vi "VersionCheck.vi"(0 "Version":string, 1 "error in (no error)":errorcluster) -> (2 "Latest Version":string, 3 "outdated?":bool, 4 "error out":errorcluster)   [LabVIEW 2024]
uses:
  <vilib>/regexp/Match Regular Expression.xnode
panel:
  out "standard output":string
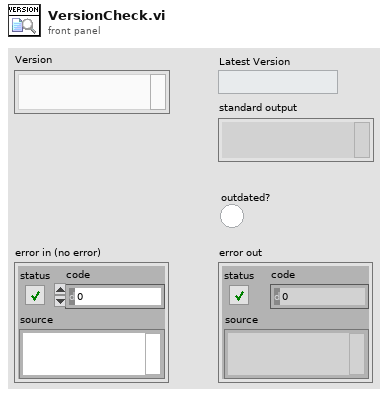
[diagram p1: front panel]
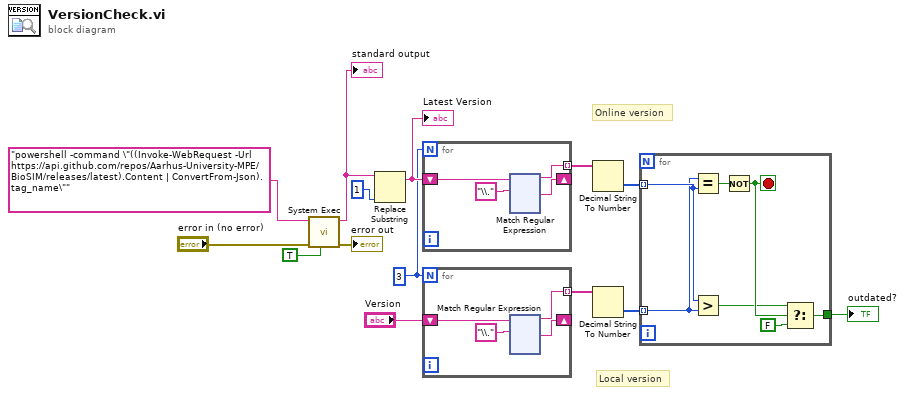
[diagram p0: block diagram]
diagram:
  w3 = 3
  # "Local version"
  # "Online version"
  n1 = call <vilib>:"System Exec.vi"("run minimized? (F)"=TRUE, "error in (no error)"="error in (no error)", "command line"="powershell -command \"((Invoke-WebRequest -Url https://api.github.com/repos/Aarhus-University-MPE/BioSIM/releases/latest).Content | ConvertFrom-Json).tag_name\"") -> ("error out"=→"error out":errorcluster, "standard output"=w12:string)  [unwired: 5 in, 2 out]
  "standard output" <- w12
  n2 = Replace Substring(2:1 ("length (len. of substring)"), 5:w12) -> (1:w10:string)  [unwired: 2 in, 1 out]
  "Latest Version" <- w10
  n3 = for {
    N: w3 -> [_]
    shift-right: [w16] -> _
    shift-left: w10 -> [w17]
    tunnel: [w15] -> w9 mode=indexing
    n4 = xnode "Match Regular Expression"("input string"=w17, "regular expression"="\\.") -> ("before match"=w15:string, "after match"=w16:string)  [unwired: 4 in, 3 out]
  }
  n5 = for {
    N: w3 -> [_]
    shift-right: [w137] -> _
    shift-left: "Version" -> [w138]
    tunnel: [w136] -> w7 mode=indexing
    n6 = xnode "Match Regular Expression"("input string"=w138, "regular expression"="\\.") -> ("before match"=w136:string, "after match"=w137:string)  [unwired: 4 in, 3 out]
  }
  n7 = Decimal String To Number(string=w9) -> (number=w8:i32[])  [unwired: 2 in, 1 out]
  n8 = Decimal String To Number(string=w7) -> (number=w5:i32[])  [unwired: 2 in, 1 out]
  n9 = for {
    tunnel: w8 -> [w262] mode=indexing
    tunnel: w5 -> [w261] mode=indexing
    tunnel: [w257] -> w4
    stop <- w260 stop-if-true
    n10 = Equal?(x=w261, y=w262) -> (x = y?=w263:bool)
    n11 = Greater?(x=w262, y=w261) -> (0:w259:bool)
    n12 = Not(x=w263) -> (.not. x?=w260:bool)
    n13 = Select(t=w259, s=w260, f=FALSE) -> (s? t:f=w257:bool)
  }
  "outdated?" <- w4
